vi "Auto Elevator Set.vi"(9 "Command":i32, 11 "Mode":i32) -> (2 "Done?":bool)   [LabVIEW 2014]
uses:
  Elevator/Elevator Control Command.ctl
  Elevator/Elevator Command.ctl
  Common Code/Elevator Mode.ctl
  Robot Global Data.vi
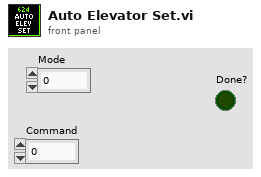
[diagram p1: front panel]
types:
  T1 = typedef "Elevator Control Command.ctl" = cluster{"Command":T2, "Manual Motor Out":dbl, "Manual Eject Piston":bool, "Mode":T3, "Override Limits":bool, "Manual Stabilizer":bool, "Manual Finger":bool, "Load from Step?":bool, "Store Trashcan?":bool}
  T2 = typedef "Elevator Command.ctl" = enum16{"Idle", "Load 1", "Load 2", "Load 3", "Drop Stack", "Eject Stack", "Load Trashcan"}
  T3 = typedef "Elevator Mode.ctl" = enum16{"Manual", "Safe", "Auto"}
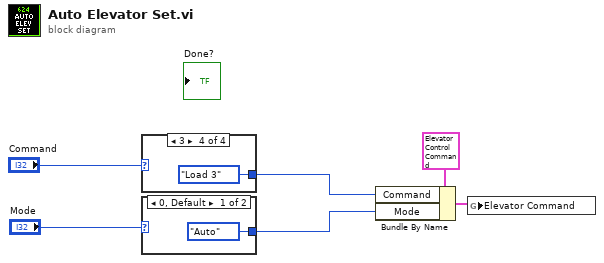
[diagram p0: block diagram]
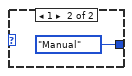
[diagram p2: hidden frame]
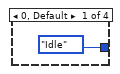
[diagram p3: hidden frame]
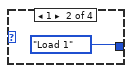
[diagram p4: hidden frame]
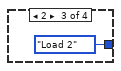
[diagram p5: hidden frame]
diagram:
  n1 = case shown="3" "Command" {
    tunnel: [Elevator_Command."Idle" ("Command") Elevator_Command."Load 1" ("Command") Elevator_Command."Load 2" ("Command") Elevator_Command."Load 3" ("Command")] -> w4
    frame 0, Default {
    }
    frame 1 {
    }
    frame 2 {
    }
    frame 3 {
    }
  }
  n2 = case shown="0, Default" "Mode" {
    tunnel: [Elevator_Mode."Auto" ("Mode") Elevator_Mode."Manual" ("Mode")] -> w3
    frame 0, Default {
    }
    frame 1 {
    }
  }
  n3 = Bundle By Name(cluster=T1 {"Command"=enum."Idle", "Manual Motor Out"=0.0, "Manual Eject Piston"=FALSE, "Mode"=enum."Manual", "Override Limits"=FALSE, "Manual Stabilizer"=FALSE, "Manual Finger"=FALSE, "Load from Step?"=FALSE, "Store Trashcan?"=FALSE} ("Elevator Command"), "Command"=w4, "Mode"=w3) -> (w6:T1)
  n4 = global write "Robot Global Data.vi" "Elevator Command"(w6) -> ()
